vi "Test_continous_unstable_weight.vi"() -> ()   [LabVIEW 2019]
panel:
  in  "Measuring interval (ms)":u32=1000
  out "Measured weight":dbl(graph)
  in  "stop\n(delay = measuring interval)":bool
  out "Double after conversion":dbl
  in  "VISA resource name":refnum<visa-resource-name>
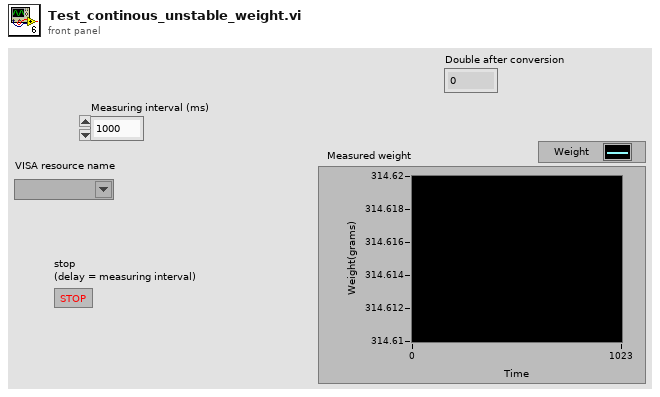
[diagram p1: front panel]
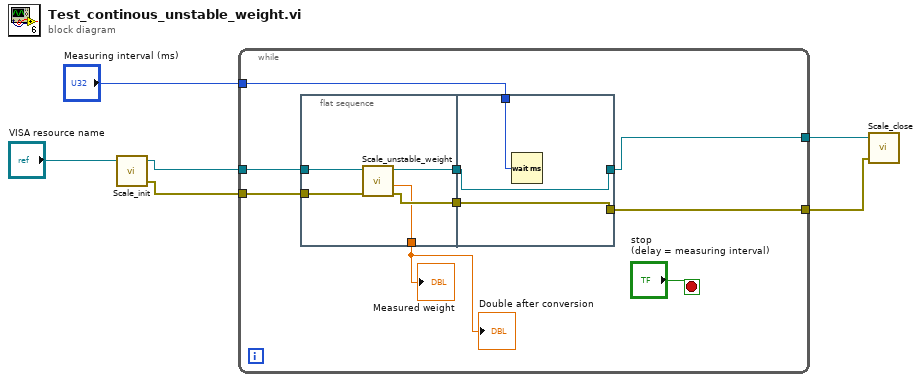
[diagram p0: block diagram]
diagram:
  n1 = call "Scale_init.vi"("VISA resource name\ncheck COM port from \ndevice manager"="VISA resource name") -> ("error out"=w4:errorcluster, "VISA resource name out"=w5:refnum<visa-resource-name>)  [unwired: 3 in]
  n2 = while {
    tunnel: w5 -> [w15]
    tunnel: w4 -> [w14]
    tunnel: [w10] -> w3
    tunnel: [w9] -> w2
    tunnel: "Measuring interval (ms)" -> [w7]
    stop <- "stop\n(delay = measuring interval)" stop-if-true
    n3 = flat-sequence {
      tunnel: w15 -> [w20]
      tunnel: w14 -> [w19]
      tunnel: [w18] -> w12
      tunnel: [w17] -> w11
      tunnel: [w16] -> w8
      tunnel: [w23] -> w10
      tunnel: w12 -> [w23]
      tunnel: [w22] -> w9
      tunnel: w11 -> [w22]
      tunnel: w7 -> [w21]
      frame #0 {
        n4 = call "Scale_unstable_weight.vi"("error in (no error)"=w19, "VISA resource name"=w20) -> ("error out"=w17:errorcluster, "Number after conversion"=w16:dbl, "VISA resource name out"=w18:refnum<visa-resource-name>)  [unwired: 2 in, 1 out]
      }
      frame #1 {
        n5 = Wait (ms)(milliseconds to wait=w21) -> ()  [unwired: 1 out]
      }
    }
    "Measured weight" <- w8
    "Double after conversion" <- w8
  }
  n6 = call "Scale_close.vi"("error in (no error)"=w2, "VISA resource name"=w3) -> ()  [unwired: 3 in, 1 out]
